vi "getAdditionalDataFromXMLNative.vi"(8 "error in (no error)":errorcluster, 10 "eventXML":refnum<k20>, 11 "RfRamp in":refnum<class "RfRamp.lvclass">) -> (0 "error out":errorcluster, 2 "eventXML out":refnum<k20>, 3 "RfRamp out":refnum<class "RfRamp.lvclass">)   [LabVIEW 2011, in "Tools.lvlib" / "Scripting.lvlib" / "RfRamp.lvclass"]
uses:
  RfRamp.lvclass
  RfRamp.lvclass/RfRamp.ctl
  <vilib>/xml/Close Reference(Node).vi
  <vilib>/xml/NI_XML.lvlib
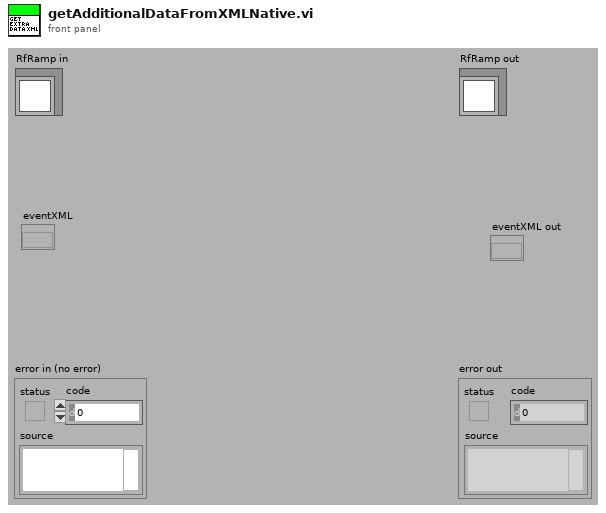
[diagram p1: front panel]
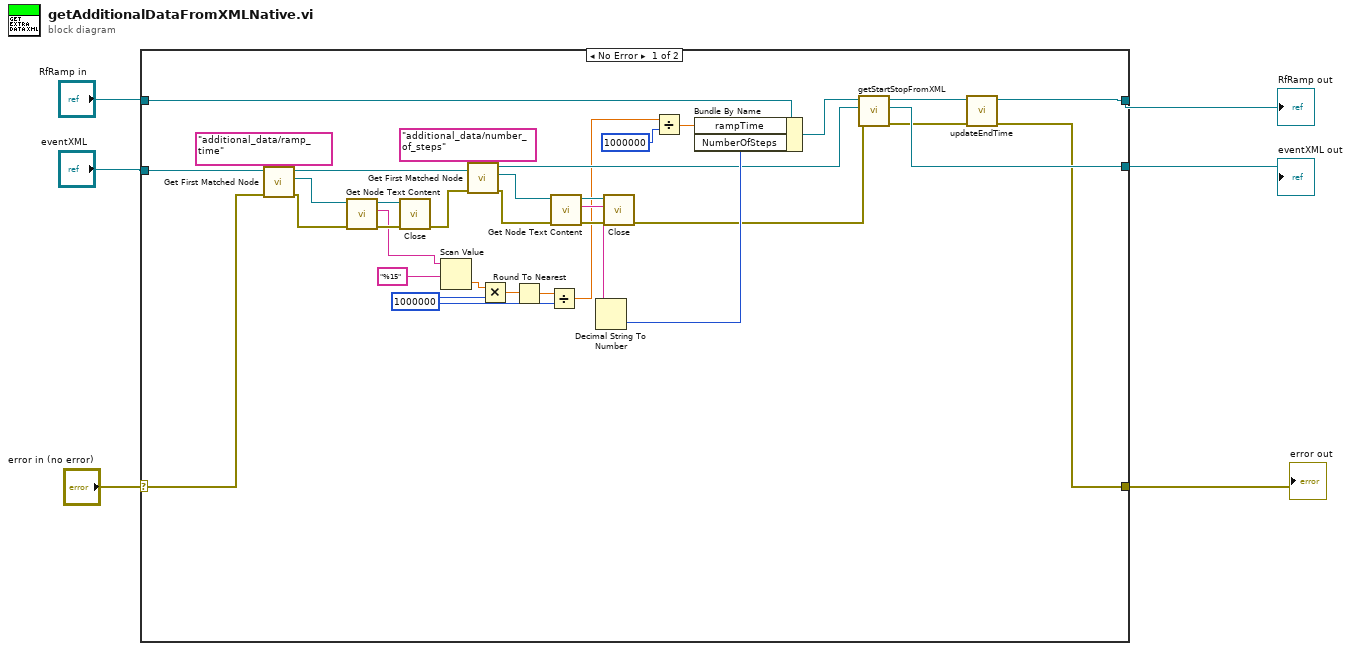
[diagram p0: block diagram]
diagram:
  n1 = case shown="No Error" "error in (no error)" {
    selector: "error in (no error)" -> [w36 w42]
    tunnel: [w14 w42] -> w2
    tunnel: [w15 w43] -> w3
    tunnel: "RfRamp in" -> [w24 w43]
    tunnel: "eventXML" -> [w37 w41]
    tunnel: [w19 w41] -> w1
    frame No Error {
      w10 = 1000000
      n2 = call <vilib>:"Get First Matched Node.vi"("error in (no error)"=w36, "XPath expression"="additional_data/ramp_time", "node in"=w37) -> ("error out"=w33:errorcluster, "node result"=w34:refnum<k20>, "node out"=w27:refnum<k20>)  [unwired: 6 in]
      n3 = call <vilib>:"Get Node Text Content.vi"("error in (no error)"=w33, "node in"=w34) -> ("error out"=w38:errorcluster, "node text"=w25:string, "node out"=w39:refnum<k20>)  [unwired: 7 in]
      n4 = call-poly <vilib>:"Close.vi"("error in (no error)"=w38, "node"=w39) -> ("error out"=w26:errorcluster)  [unwired: 7 in]
      n5 = Scan Value(string=w25, format string="%15") -> (value=w13:dbl)  [unwired: 1 in, 1 out]
      n6 = call <vilib>:"Get First Matched Node.vi"("error in (no error)"=w26, "XPath expression"="additional_data/number_of_steps", "node in"=w27) -> ("error out"=w32:errorcluster, "node result"=w31:refnum<k20>, "node out"=w20:refnum<k20>)  [unwired: 6 in]
      n7 = Multiply(x=w13, y=w10) -> (x*y=w12:dbl)
      n8 = Round To Nearest(number=w12) -> (nearest integer value=w11:dbl)
      n9 = Divide(x=w11, y=w10) -> (x/y=w8:dbl)
      n10 = call <vilib>:"Get Node Text Content.vi"("error in (no error)"=w32, "node in"=w31) -> ("error out"=w29:errorcluster, "node text"=w23:string, "node out"=w28:refnum<k20>)  [unwired: 7 in]
      n11 = Decimal String To Number(string=w23) -> (number=w22:i32)  [unwired: 2 in, 1 out]
      n12 = call-poly <vilib>:"Close.vi"("error in (no error)"=w29, "node"=w28) -> ("error out"=w18:errorcluster)  [unwired: 7 in]
      n13 = Divide(x=w8, y=1000000) -> (x/y=w9:dbl)
      n14 = Bundle By Name(cluster=w24, "rampTime"=w9, "NumberOfSteps"=w22) -> (w21:refnum<class "RfRamp.lvclass">)
      n15 = call "getStartStopFromXML.vi"("error in (no error)"=w18, "eventXML"=w20, "RfRamp in"=w21) -> ("error out"=w16:errorcluster, "eventXML out"=w19:refnum<k20>, "RfRamp out"=w17:refnum<class "RfRamp.lvclass">)  [unwired: 6 in]
      n16 = call-dynamic "updateEndTime.vi"("error in (no error)"=w16, "RfRamp in"=w17) -> ("error out"=w14:errorcluster, "RfRamp out"=w15:refnum<class "RfRamp.lvclass">)  [unwired: 8 in]
    }
    frame Error {
    }
  }
  "error out" <- w2
  "RfRamp out" <- w3
  "eventXML out" <- w1
